vi "输入数据解析.vi"(0 "单个参数补充":dbl, 1 "从板号":dbl=1.0, 2 "主板二维码":string="BNET01", 3 "从板二维码":string="BNET01", 5 "主板引用":refnum<vi>, 7 "从板引用":refnum<vi>, 9 "主板选项":string="三级故障阀值", 11 "枚举":enum16{"主板", "从板"}(ring), 12 "快换":bool caption="快换写入") -> (4 "输出数组":dbl[][](array[numeric]), 6 "数组长度":dbl[](array[numeric]), 8 "循环次数":i32, 10 "命令":u32, 14 "名称":string[](array[string]), 15 "命令序号":u32[](array[numeric]))   [LabVIEW 2013] (continued)
                    n7569 = Quotient & Remainder(x=w19481, y=w19499) -> (x-y*floor(x/y)=w19498:dbl, floor(x/y)=w19502:dbl)
                    n7570 = Quotient & Remainder(x=w19480, y=w19494) -> (x-y*floor(x/y)=w19490:dbl, floor(x/y)=w19491:dbl)
                    n7571 = Quotient & Remainder(x=w19502, y=w19499) -> (x-y*floor(x/y)=w19497:dbl, floor(x/y)=w19501:dbl)
                    n7572 = Quotient & Remainder(x=w19491, y=w19494) -> (x-y*floor(x/y)=w19489:dbl, floor(x/y)=w19492:dbl)
                    n7573 = Quotient & Remainder(x=w19501, y=w19499) -> (x-y*floor(x/y)=w19496:dbl, floor(x/y)=w19500:dbl)
                    n7574 = Quotient & Remainder(x=w19492, y=w19494) -> (x-y*floor(x/y)=w19488:dbl, floor(x/y)=w19493:dbl)
                    n7575 = Quotient & Remainder(x=w19500, y=w19499) -> (x-y*floor(x/y)=w19495:dbl)  [unwired: 1 out]
                    n7576 = Quotient & Remainder(x=w19493, y=w19494) -> (x-y*floor(x/y)=w19487:dbl)  [unwired: 1 out]
                    n7577 = Build Array(w19495, w19496, w19497, w19498, w19487, w19488, w19489, w19490) -> (w19503:dbl[])
                  }
                  frame 3 {
                    w19511 = 256.0 ("y")
                    # "充电次数"
                    n7578 = Unbundle By Name(w19516) -> ("充电次数"=w19515:dbl, "应用车型"=w19513:dbl, "电池包组号"=w19512:dbl)
                    n7579 = Quotient & Remainder(x=w19515, y=w19511) -> (x-y*floor(x/y)=w19517:dbl, floor(x/y)=w19514:dbl)
                    n7580 = Quotient & Remainder(x=w19513, y=w19511) -> (x-y*floor(x/y)=w19509:dbl, floor(x/y)=w19510:dbl)
                    n7581 = Quotient & Remainder(x=w19512, y=w19511) -> (x-y*floor(x/y)=w19507:dbl, floor(x/y)=w19508:dbl)
                    n7582 = Build Array(w19514, w19517, w19510, w19509, w19508, w19507) -> (w19518:dbl[])
                  }
                  frame 4 {
                    # "SOC"
                    n7583 = Unbundle By Name(w19527) -> ("SOC"=w19526:dbl)
                    n7584 = call "输入分辨率计算-EV05.vi"("1字节?"=FALSE, "数值"=w19526, "分辨率"=0.1) -> ("低字节"=w19522:dbl, "高字节1"=w19523:dbl)  [unwired: 2 in, 5 out]
                    n7585 = Build Array(w19523, w19522) -> (w19528:dbl[])
                  }
                  frame 5 {
                    # "车牌号"
                    n7586 = Unbundle By Name(w19535) -> ("车牌号"=w19534:string)
                    n7587 = String To Byte Array(string=w19534) -> (unsigned byte array=w19538:u8[])
                    n7588 = Array Subset(array=w19538, length=8 ("长度")) -> (w19533:u8[])  [unwired: 1 in]
                  }
                  frame 6 {
                    n7589 = Unbundle By Name(w19556) -> ("最大允许单体电压"=w19554:dbl, "最大允许总电压"=w19553:dbl, "最大允许温度"=w19552:dbl, "最小允许温度"=w19551:dbl, "最大允许充电电流"=w19550:dbl, "最小允许充电电流"=w19549:dbl, "电流步长"=w19545:dbl, "最小允许单体电压"=w19548:dbl)
                    n7590 = call "输入分辨率计算-EV05.vi"("1字节?"=FALSE, "数值 2"=w19548, "数值"=w19554, "分辨率"=0.001) -> ("低字节 2"=w19540:dbl, "高字节 2"=w19541:dbl, "低字节"=w19564:dbl, "高字节1"=w19565:dbl)  [unwired: 1 in, 3 out]
                    n7591 = call "输入分辨率计算-EV05.vi"("1字节?"=FALSE, "数值"=w19553, "分辨率"=0.1) -> ("低字节"=w19562:dbl, "高字节1"=w19563:dbl)  [unwired: 2 in, 5 out]
                    n7592 = call "输入分辨率计算-EV05.vi"("1字节?"=TRUE, "数值 2"=w19551, "数值"=w19552, "偏移量"=-40.0, "分辨率"=1.0) -> ("高字节 2"=w19557:dbl, "高字节1"=w19561:dbl)  [unwired: 5 out]
                    n7593 = call "输入分辨率计算-EV05.vi"("1字节?"=FALSE, "数值 2"=w19549, "数值"=w19550, "偏移量"=0.0, "分辨率"=0.1) -> ("低字节 2"=w19546:dbl, "高字节 2"=w19547:dbl, "低字节"=w19559:dbl, "高字节1"=w19560:dbl)  [unwired: 3 out]
                    n7594 = Quotient & Remainder(x=w19545, y=256.0) -> (x-y*floor(x/y)=w19542:dbl, floor(x/y)=w19543:dbl)
                    n7595 = Build Array(w19565, w19564, w19563, w19562, w19561, w19557, w19560, w19559, w19547, w19546, w19543, w19542, w19541, w19540) -> (w19558:dbl[])
                  }
                }
              }
            }
          }
        }
        frame "电池包序号" {
          n7596 = case shown="真" w19580 {
            tunnel: [_ w19591] -> w19584
            tunnel: [_ w19590] -> w19583
            tunnel: w19582 -> [_ w19586]
            tunnel: [_ w19589] -> w19581
            tunnel: [_ u32 35 ("命令序号")] -> w19579
            frame False {
            }
            frame True {
              n7597 = Unbundle By Name(w19586) -> ("电池组信息(从板)"=w19587:refnum<vi>)
              n7598 = property class="Clust (严格)"(reference=w19587) -> ("Value"=w19585:T9)  [unwired: 1 in, 2 out]
              n7599 = for {
                N: 1 -> [_]
                tunnel: [w19597] -> w19591 mode=indexing
                tunnel: [w19596] -> w19590 mode=indexing
                tunnel: w19585 -> [w19595]
                tunnel: [w19594] -> w19589 mode=indexing
                i -> [w19593]
                n7600 = case shown="0, 默认" w19593 {
                  tunnel: [4 ("单个参数补充") 30 ("单个参数补充") 8 ("单个参数补充") 6 ("单个参数补充") 4 ("单个参数补充") 8 ("单个参数补充") 14 ("单个参数补充")] -> w19597
                  tunnel: [u32 2 ("命令序号") u32 1 ("命令序号") u32 3 ("命令序号") u32 4 ("命令序号") u32 5 ("命令序号") u32 6 ("命令序号") u32 7 ("命令序号")] -> w19596
                  tunnel: w19595 -> [w19605 w19621 w19633 w19662 w19672 w19679 w19699]
                  tunnel: [w19598 w19623 w19650 w19664 w19673 w19677 w19701] -> w19594
                  frame 0, Default {
                    n7601 = Unbundle By Name(w19605) -> ("电池包序号"=w19602:dbl)
                    n7602 = Quotient & Remainder(x=w19602, y=256.0) -> (x-y*floor(x/y)=w19599:dbl, floor(x/y)=w19600:dbl)
                    n7603 = Build Array(w19600, w19599) -> (w19598:dbl[])
                  }
                  frame 1 {
                    w19611 = 0 ("索引")
                    # "电池组信息"
                    n7604 = Unbundle By Name(w19621) -> ("电池类型"=w19613:dbl, "电池厂家"=w19612:dbl, "电池厂家"=w19614:dbl, "电池类型"=w19615:dbl, "额定能量"=w19619:dbl, "额定容量"=w19616:dbl, "实际容量"=w19608:dbl)
                    n7605 = Build Array(w19613, w19612, w19611, w19611, w19611, w19611, w19611, w19614, w19615) -> (w19610:dbl[])
                    n7606 = call "输入分辨率计算-EV05.vi"("1字节?"=FALSE, "数值"=w19608, "分辨率"=0.1) -> ("高字节1"=w19606:dbl)  [unwired: 2 in, 6 out]
                    n7607 = Quotient & Remainder(x=w19619, y=256.0) -> (x-y*floor(x/y)=w19617:dbl, floor(x/y)=w19618:dbl)
                    n7608 = call "电池组信息组合.vi"("数组"=w19610) -> ("电池信息组合"=w19624:dbl[])
                    n7609 = Insert Into Array(array=w19624, index=0 ("索引"), new element #1=w19618, new element #2=w19617, new element #3=w19616, new element #4=w19606, new element #5=w19606) -> (w19623:dbl[])
                  }
                  frame 2 {
                    w19641 = 256.0 ("y")
                    w19646 = 256.0 ("y")
                    # "充放电安时/安时数"
                    n7610 = Unbundle By Name(w19633) -> ("充电总安时"=w19630:dbl, "放电总这时"=w19629:dbl)
                    n7611 = call "输入分辨率计算-EV05.vi"("1字节?"=TRUE, "数值 2"=w19629, "数值"=w19630, "分辨率"=0.001) -> ("高字节 2"=w19627:dbl, "高字节1"=w19628:dbl)  [unwired: 1 in, 5 out]
                    n7612 = Quotient & Remainder(x=w19628, y=w19646) -> (x-y*floor(x/y)=w19645:dbl, floor(x/y)=w19649:dbl)
                    n7613 = Quotient & Remainder(x=w19627, y=w19641) -> (x-y*floor(x/y)=w19637:dbl, floor(x/y)=w19638:dbl)
                    n7614 = Quotient & Remainder(x=w19649, y=w19646) -> (x-y*floor(x/y)=w19644:dbl, floor(x/y)=w19648:dbl)
                    n7615 = Quotient & Remainder(x=w19638, y=w19641) -> (x-y*floor(x/y)=w19636:dbl, floor(x/y)=w19639:dbl)
                    n7616 = Quotient & Remainder(x=w19648, y=w19646) -> (x-y*floor(x/y)=w19643:dbl, floor(x/y)=w19647:dbl)
                    n7617 = Quotient & Remainder(x=w19639, y=w19641) -> (x-y*floor(x/y)=w19635:dbl, floor(x/y)=w19640:dbl)
                    n7618 = Quotient & Remainder(x=w19647, y=w19646) -> (x-y*floor(x/y)=w19642:dbl)  [unwired: 1 out]
                    n7619 = Quotient & Remainder(x=w19640, y=w19641) -> (x-y*floor(x/y)=w19634:dbl)  [unwired: 1 out]
                    n7620 = Build Array(w19642, w19643, w19644, w19645, w19634, w19635, w19636, w19637) -> (w19650:dbl[])
                  }
                  frame 3 {
                    w19657 = 256.0 ("y")
                    # "充电次数"
                    n7621 = Unbundle By Name(w19662) -> ("充电次数"=w19661:dbl, "应用车型"=w19659:dbl, "电池包组号"=w19658:dbl)
                    n7622 = Quotient & Remainder(x=w19661, y=w19657) -> (x-y*floor(x/y)=w19663:dbl, floor(x/y)=w19660:dbl)
                    n7623 = Quotient & Remainder(x=w19659, y=w19657) -> (x-y*floor(x/y)=w19655:dbl, floor(x/y)=w19656:dbl)
                    n7624 = Quotient & Remainder(x=w19658, y=w19657) -> (x-y*floor(x/y)=w19653:dbl, floor(x/y)=w19654:dbl)
                    n7625 = Build Array(w19660, w19663, w19656, w19655, w19654, w19653) -> (w19664:dbl[])
                  }
                  frame 4 {
                    # "SOC"
                    n7626 = Unbundle By Name(w19672) -> ("SOC"=w19671:dbl)
                    n7627 = call "输入分辨率计算-EV05.vi"("1字节?"=FALSE, "数值"=w19671, "分辨率"=0.1) -> ("低字节"=w19667:dbl, "高字节1"=w19668:dbl)  [unwired: 2 in, 5 out]
                    n7628 = Build Array(w19668, w19667) -> (w19673:dbl[])
                  }
                  frame 5 {
                    # "车牌号"
                    n7629 = Unbundle By Name(w19679) -> ("车牌号"=w19678:string)
                    n7630 = String To Byte Array(string=w19678) -> (unsigned byte array=w19682:u8[])
                    n7631 = Array Subset(array=w19682, length=8 ("长度")) -> (w19677:u8[])  [unwired: 1 in]
                  }
                  frame 6 {
                    n7632 = Unbundle By Name(w19699) -> ("最大允许单体电压"=w19697:dbl, "最大允许总电压"=w19696:dbl, "最大允许温度"=w19695:dbl, "最小允许温度"=w19694:dbl, "最大允许充电电流"=w19693:dbl, "最小允许充电电流"=w19692:dbl, "电流步长"=w19688:dbl, "最小允许单体电压"=w19691:dbl)
                    n7633 = call "输入分辨率计算-EV05.vi"("1字节?"=FALSE, "数值 2"=w19691, "数值"=w19697, "分辨率"=0.001) -> ("低字节 2"=w19683:dbl, "高字节 2"=w19684:dbl, "低字节"=w19707:dbl, "高字节1"=w19708:dbl)  [unwired: 1 in, 3 out]
                    n7634 = call "输入分辨率计算-EV05.vi"("1字节?"=FALSE, "数值"=w19696, "分辨率"=0.1) -> ("低字节"=w19705:dbl, "高字节1"=w19706:dbl)  [unwired: 2 in, 5 out]
                    n7635 = call "输入分辨率计算-EV05.vi"("1字节?"=TRUE, "数值 2"=w19694, "数值"=w19695, "偏移量"=-40.0, "分辨率"=1.0) -> ("高字节 2"=w19700:dbl, "高字节1"=w19704:dbl)  [unwired: 5 out]
                    n7636 = call "输入分辨率计算-EV05.vi"("1字节?"=FALSE, "数值 2"=w19692, "数值"=w19693, "偏移量"=0.0, "分辨率"=0.1) -> ("低字节 2"=w19689:dbl, "高字节 2"=w19690:dbl, "低字节"=w19702:dbl, "高字节1"=w19703:dbl)  [unwired: 3 out]
                    n7637 = Quotient & Remainder(x=w19688, y=256.0) -> (x-y*floor(x/y)=w19685:dbl, floor(x/y)=w19686:dbl)
                    n7638 = Build Array(w19708, w19707, w19706, w19705, w19704, w19700, w19703, w19702, w19690, w19689, w19686, w19685, w19684, w19683) -> (w19701:dbl[])
                  }
                }
              }
            }
          }
        }
        frame "充放电安时" {
          n7639 = case shown="真" w19723 {
            tunnel: [_ w19734] -> w19727
            tunnel: [_ w19733] -> w19726
            tunnel: w19725 -> [_ w19729]
            tunnel: [_ w19732] -> w19724
            tunnel: [_ u32 35 ("命令序号")] -> w19722
            frame False {
            }
            frame True {
              n7640 = Unbundle By Name(w19729) -> ("电池组信息(从板)"=w19730:refnum<vi>)
              n7641 = property class="Clust (严格)"(reference=w19730) -> ("Value"=w19728:T9)  [unwired: 1 in, 2 out]
              n7642 = for {
                N: 1 -> [_]
                tunnel: [w19740] -> w19734 mode=indexing
                tunnel: [w19739] -> w19733 mode=indexing
                tunnel: w19728 -> [w19738]
                tunnel: [w19737] -> w19732 mode=indexing
                i -> [w19736]
                n7643 = case shown="0, 默认" w19736 {
                  tunnel: [8 ("单个参数补充") 30 ("单个参数补充") 4 ("单个参数补充") 6 ("单个参数补充") 4 ("单个参数补充") 8 ("单个参数补充") 14 ("单个参数补充")] -> w19740
                  tunnel: [u32 3 ("命令序号") u32 1 ("命令序号") u32 2 ("命令序号") u32 4 ("命令序号") u32 5 ("命令序号") u32 6 ("命令序号") u32 7 ("命令序号")] -> w19739
                  tunnel: w19738 -> [w19747 w19782 w19795 w19805 w19815 w19822 w19842]
                  tunnel: [w19764 w19784 w19788 w19807 w19816 w19820 w19844] -> w19737
                  frame 0, Default {
                    w19755 = 256.0 ("y")
                    w19760 = 256.0 ("y")
                    # "充放电安时/安时数"
                    n7644 = Unbundle By Name(w19747) -> ("充电总安时"=w19744:dbl, "放电总这时"=w19743:dbl)
                    n7645 = call "输入分辨率计算-EV05.vi"("1字节?"=TRUE, "数值 2"=w19743, "数值"=w19744, "分辨率"=0.001) -> ("高字节 2"=w19741:dbl, "高字节1"=w19742:dbl)  [unwired: 1 in, 5 out]
                    n7646 = Quotient & Remainder(x=w19742, y=w19760) -> (x-y*floor(x/y)=w19759:dbl, floor(x/y)=w19763:dbl)
                    n7647 = Quotient & Remainder(x=w19741, y=w19755) -> (x-y*floor(x/y)=w19751:dbl, floor(x/y)=w19752:dbl)
                    n7648 = Quotient & Remainder(x=w19763, y=w19760) -> (x-y*floor(x/y)=w19758:dbl, floor(x/y)=w19762:dbl)
                    n7649 = Quotient & Remainder(x=w19752, y=w19755) -> (x-y*floor(x/y)=w19750:dbl, floor(x/y)=w19753:dbl)
                    n7650 = Quotient & Remainder(x=w19762, y=w19760) -> (x-y*floor(x/y)=w19757:dbl, floor(x/y)=w19761:dbl)
                    n7651 = Quotient & Remainder(x=w19753, y=w19755) -> (x-y*floor(x/y)=w19749:dbl, floor(x/y)=w19754:dbl)
                    n7652 = Quotient & Remainder(x=w19761, y=w19760) -> (x-y*floor(x/y)=w19756:dbl)  [unwired: 1 out]
                    n7653 = Quotient & Remainder(x=w19754, y=w19755) -> (x-y*floor(x/y)=w19748:dbl)  [unwired: 1 out]
                    n7654 = Build Array(w19756, w19757, w19758, w19759, w19748, w19749, w19750, w19751) -> (w19764:dbl[])
                  }
                  frame 1 {
                    w19772 = 0 ("索引")
                    # "电池组信息"
                    n7655 = Unbundle By Name(w19782) -> ("电池类型"=w19774:dbl, "电池厂家"=w19773:dbl, "电池厂家"=w19775:dbl, "电池类型"=w19776:dbl, "额定能量"=w19780:dbl, "额定容量"=w19777:dbl, "实际容量"=w19769:dbl)
                    n7656 = Build Array(w19774, w19773, w19772, w19772, w19772, w19772, w19772, w19775, w19776) -> (w19771:dbl[])
                    n7657 = call "输入分辨率计算-EV05.vi"("1字节?"=FALSE, "数值"=w19769, "分辨率"=0.1) -> ("高字节1"=w19767:dbl)  [unwired: 2 in, 6 out]
                    n7658 = Quotient & Remainder(x=w19780, y=256.0) -> (x-y*floor(x/y)=w19778:dbl, floor(x/y)=w19779:dbl)
                    n7659 = call "电池组信息组合.vi"("数组"=w19771) -> ("电池信息组合"=w19785:dbl[])
                    n7660 = Insert Into Array(array=w19785, index=0 ("索引"), new element #1=w19779, new element #2=w19778, new element #3=w19777, new element #4=w19767, new element #5=w19767) -> (w19784:dbl[])
                  }
                  frame 2 {
                    n7661 = Unbundle By Name(w19795) -> ("电池包序号"=w19792:dbl)
                    n7662 = Quotient & Remainder(x=w19792, y=256.0) -> (x-y*floor(x/y)=w19789:dbl, floor(x/y)=w19790:dbl)
                    n7663 = Build Array(w19790, w19789) -> (w19788:dbl[])
                  }
                  frame 3 {
                    w19800 = 256.0 ("y")
                    # "充电次数"
                    n7664 = Unbundle By Name(w19805) -> ("充电次数"=w19804:dbl, "应用车型"=w19802:dbl, "电池包组号"=w19801:dbl)
                    n7665 = Quotient & Remainder(x=w19804, y=w19800) -> (x-y*floor(x/y)=w19806:dbl, floor(x/y)=w19803:dbl)
                    n7666 = Quotient & Remainder(x=w19802, y=w19800) -> (x-y*floor(x/y)=w19798:dbl, floor(x/y)=w19799:dbl)
                    n7667 = Quotient & Remainder(x=w19801, y=w19800) -> (x-y*floor(x/y)=w19796:dbl, floor(x/y)=w19797:dbl)
                    n7668 = Build Array(w19803, w19806, w19799, w19798, w19797, w19796) -> (w19807:dbl[])
                  }
                  frame 4 {
                    # "SOC"
                    n7669 = Unbundle By Name(w19815) -> ("SOC"=w19814:dbl)
                    n7670 = call "输入分辨率计算-EV05.vi"("1字节?"=FALSE, "数值"=w19814, "分辨率"=0.1) -> ("低字节"=w19810:dbl, "高字节1"=w19811:dbl)  [unwired: 2 in, 5 out]
                    n7671 = Build Array(w19811, w19810) -> (w19816:dbl[])
                  }
                  frame 5 {
                    # "车牌号"
                    n7672 = Unbundle By Name(w19822) -> ("车牌号"=w19821:string)
                    n7673 = String To Byte Array(string=w19821) -> (unsigned byte array=w19825:u8[])
                    n7674 = Array Subset(array=w19825, length=8 ("长度")) -> (w19820:u8[])  [unwired: 1 in]
                  }
                  frame 6 {
                    n7675 = Unbundle By Name(w19842) -> ("最大允许单体电压"=w19840:dbl, "最大允许总电压"=w19839:dbl, "最大允许温度"=w19838:dbl, "最小允许温度"=w19837:dbl, "最大允许充电电流"=w19836:dbl, "最小允许充电电流"=w19835:dbl, "电流步长"=w19831:dbl, "最小允许单体电压"=w19834:dbl)
                    n7676 = call "输入分辨率计算-EV05.vi"("1字节?"=FALSE, "数值 2"=w19834, "数值"=w19840, "分辨率"=0.001) -> ("低字节 2"=w19826:dbl, "高字节 2"=w19827:dbl, "低字节"=w19850:dbl, "高字节1"=w19851:dbl)  [unwired: 1 in, 3 out]
                    n7677 = call "输入分辨率计算-EV05.vi"("1字节?"=FALSE, "数值"=w19839, "分辨率"=0.1) -> ("低字节"=w19848:dbl, "高字节1"=w19849:dbl)  [unwired: 2 in, 5 out]
                    n7678 = call "输入分辨率计算-EV05.vi"("1字节?"=TRUE, "数值 2"=w19837, "数值"=w19838, "偏移量"=-40.0, "分辨率"=1.0) -> ("高字节 2"=w19843:dbl, "高字节1"=w19847:dbl)  [unwired: 5 out]
                    n7679 = call "输入分辨率计算-EV05.vi"("1字节?"=FALSE, "数值 2"=w19835, "数值"=w19836, "偏移量"=0.0, "分辨率"=0.1) -> ("低字节 2"=w19832:dbl, "高字节 2"=w19833:dbl, "低字节"=w19845:dbl, "高字节1"=w19846:dbl)  [unwired: 3 out]
                    n7680 = Quotient & Remainder(x=w19831, y=256.0) -> (x-y*floor(x/y)=w19828:dbl, floor(x/y)=w19829:dbl)
                    n7681 = Build Array(w19851, w19850, w19849, w19848, w19847, w19843, w19846, w19845, w19833, w19832, w19829, w19828, w19827, w19826) -> (w19844:dbl[])
                  }
                }
              }
            }
          }
        }
        frame "充电次数时间" {
          n7682 = case shown="真" w19866 {
            tunnel: [_ w19877] -> w19870
            tunnel: [_ w19876] -> w19869
            tunnel: w19868 -> [_ w19872]
            tunnel: [_ w19875] -> w19867
            tunnel: [_ u32 35 ("命令序号")] -> w19865
            frame False {
            }
            frame True {
              n7683 = Unbundle By Name(w19872) -> ("电池组信息(从板)"=w19873:refnum<vi>)
              n7684 = property class="Clust (严格)"(reference=w19873) -> ("Value"=w19871:T9)  [unwired: 1 in, 2 out]
              n7685 = for {
                N: 1 -> [_]
                tunnel: [w19883] -> w19877 mode=indexing
                tunnel: [w19882] -> w19876 mode=indexing
                tunnel: w19871 -> [w19881]
                tunnel: [w19880] -> w19875 mode=indexing
                i -> [w19879]
                n7686 = case shown="0, 默认" w19879 {
                  tunnel: [6 ("单个参数补充") 30 ("单个参数补充") 4 ("单个参数补充") 8 ("单个参数补充") 4 ("单个参数补充") 8 ("单个参数补充") 14 ("单个参数补充")] -> w19883
                  tunnel: [u32 4 ("命令序号") u32 1 ("命令序号") u32 2 ("命令序号") u32 3 ("命令序号") u32 5 ("命令序号") u32 6 ("命令序号") u32 7 ("命令序号")] -> w19882
                  tunnel: w19881 -> [w19893 w19913 w19926 w19933 w19958 w19965 w19985]
                  tunnel: [w19895 w19915 w19919 w19950 w19959 w19963 w19987] -> w19880
                  frame 0, Default {
                    w19888 = 256.0 ("y")
                    # "充电次数"
                    n7687 = Unbundle By Name(w19893) -> ("放空次数"=w19892:dbl, "充满次数"=w19890:dbl, "充电次数"=w19889:dbl)
                    n7688 = Quotient & Remainder(x=w19892, y=w19888) -> (x-y*floor(x/y)=w19894:dbl, floor(x/y)=w19891:dbl)
                    n7689 = Quotient & Remainder(x=w19890, y=w19888) -> (x-y*floor(x/y)=w19886:dbl, floor(x/y)=w19887:dbl)
                    n7690 = Quotient & Remainder(x=w19889, y=w19888) -> (x-y*floor(x/y)=w19884:dbl, floor(x/y)=w19885:dbl)
                    n7691 = Build Array(w19891, w19894, w19887, w19886, w19885, w19884) -> (w19895:dbl[])
                  }
                  frame 1 {
                    w19903 = 0 ("索引")
                    # "电池组信息"
                    n7692 = Unbundle By Name(w19913) -> ("电池类型"=w19905:dbl, "电池厂家"=w19904:dbl, "电池厂家"=w19906:dbl, "电池类型"=w19907:dbl, "额定能量"=w19911:dbl, "额定容量"=w19908:dbl, "实际容量"=w19900:dbl)
                    n7693 = Build Array(w19905, w19904, w19903, w19903, w19903, w19903, w19903, w19906, w19907) -> (w19902:dbl[])
                    n7694 = call "输入分辨率计算-EV05.vi"("1字节?"=FALSE, "数值"=w19900, "分辨率"=0.1) -> ("高字节1"=w19898:dbl)  [unwired: 2 in, 6 out]
                    n7695 = Quotient & Remainder(x=w19911, y=256.0) -> (x-y*floor(x/y)=w19909:dbl, floor(x/y)=w19910:dbl)
                    n7696 = call "电池组信息组合.vi"("数组"=w19902) -> ("电池信息组合"=w19916:dbl[])
                    n7697 = Insert Into Array(array=w19916, index=0 ("索引"), new element #1=w19910, new element #2=w19909, new element #3=w19908, new element #4=w19898, new element #5=w19898) -> (w19915:dbl[])
                  }
                  frame 2 {
                    n7698 = Unbundle By Name(w19926) -> ("电池包序号"=w19923:dbl)
                    n7699 = Quotient & Remainder(x=w19923, y=256.0) -> (x-y*floor(x/y)=w19920:dbl, floor(x/y)=w19921:dbl)
                    n7700 = Build Array(w19921, w19920) -> (w19919:dbl[])
                  }
                  frame 3 {
                    w19941 = 256.0 ("y")
                    w19946 = 256.0 ("y")
                    # "充放电安时/安时数"
                    n7701 = Unbundle By Name(w19933) -> ("充电总安时"=w19930:dbl, "放电总这时"=w19929:dbl)
                    n7702 = call "输入分辨率计算-EV05.vi"("1字节?"=TRUE, "数值 2"=w19929, "数值"=w19930, "分辨率"=0.001) -> ("高字节 2"=w19927:dbl, "高字节1"=w19928:dbl)  [unwired: 1 in, 5 out]
                    n7703 = Quotient & Remainder(x=w19928, y=w19946) -> (x-y*floor(x/y)=w19945:dbl, floor(x/y)=w19949:dbl)
                    n7704 = Quotient & Remainder(x=w19927, y=w19941) -> (x-y*floor(x/y)=w19937:dbl, floor(x/y)=w19938:dbl)
                    n7705 = Quotient & Remainder(x=w19949, y=w19946) -> (x-y*floor(x/y)=w19944:dbl, floor(x/y)=w19948:dbl)
                    n7706 = Quotient & Remainder(x=w19938, y=w19941) -> (x-y*floor(x/y)=w19936:dbl, floor(x/y)=w19939:dbl)
                    n7707 = Quotient & Remainder(x=w19948, y=w19946) -> (x-y*floor(x/y)=w19943:dbl, floor(x/y)=w19947:dbl)
                    n7708 = Quotient & Remainder(x=w19939, y=w19941) -> (x-y*floor(x/y)=w19935:dbl, floor(x/y)=w19940:dbl)
                    n7709 = Quotient & Remainder(x=w19947, y=w19946) -> (x-y*floor(x/y)=w19942:dbl)  [unwired: 1 out]
                    n7710 = Quotient & Remainder(x=w19940, y=w19941) -> (x-y*floor(x/y)=w19934:dbl)  [unwired: 1 out]
                    n7711 = Build Array(w19942, w19943, w19944, w19945, w19934, w19935, w19936, w19937) -> (w19950:dbl[])
                  }
                  frame 4 {
                    # "SOC"
                    n7712 = Unbundle By Name(w19958) -> ("SOC"=w19957:dbl)
                    n7713 = call "输入分辨率计算-EV05.vi"("1字节?"=FALSE, "数值"=w19957, "分辨率"=0.1) -> ("低字节"=w19953:dbl, "高字节1"=w19954:dbl)  [unwired: 2 in, 5 out]
                    n7714 = Build Array(w19954, w19953) -> (w19959:dbl[])
                  }
                  frame 5 {
                    # "车牌号"
                    n7715 = Unbundle By Name(w19965) -> ("车牌号"=w19964:string)
                    n7716 = String To Byte Array(string=w19964) -> (unsigned byte array=w19968:u8[])
                    n7717 = Array Subset(array=w19968, length=8 ("长度")) -> (w19963:u8[])  [unwired: 1 in]
                  }
                  frame 6 {
                    n7718 = Unbundle By Name(w19985) -> ("最大允许单体电压"=w19983:dbl, "最大允许总电压"=w19982:dbl, "最大允许温度"=w19981:dbl, "最小允许温度"=w19980:dbl, "最大允许充电电流"=w19979:dbl, "最小允许充电电流"=w19978:dbl, "电流步长"=w19974:dbl, "最小允许单体电压"=w19977:dbl)
                    n7719 = call "输入分辨率计算-EV05.vi"("1字节?"=FALSE, "数值 2"=w19977, "数值"=w19983, "分辨率"=0.001) -> ("低字节 2"=w19969:dbl, "高字节 2"=w19970:dbl, "低字节"=w19993:dbl, "高字节1"=w19994:dbl)  [unwired: 1 in, 3 out]
                    n7720 = call "输入分辨率计算-EV05.vi"("1字节?"=FALSE, "数值"=w19982, "分辨率"=0.1) -> ("低字节"=w19991:dbl, "高字节1"=w19992:dbl)  [unwired: 2 in, 5 out]
                    n7721 = call "输入分辨率计算-EV05.vi"("1字节?"=TRUE, "数值 2"=w19980, "数值"=w19981, "偏移量"=-40.0, "分辨率"=1.0) -> ("高字节 2"=w19986:dbl, "高字节1"=w19990:dbl)  [unwired: 5 out]
                    n7722 = call "输入分辨率计算-EV05.vi"("1字节?"=FALSE, "数值 2"=w19978, "数值"=w19979, "偏移量"=0.0, "分辨率"=0.1) -> ("低字节 2"=w19975:dbl, "高字节 2"=w19976:dbl, "低字节"=w19988:dbl, "高字节1"=w19989:dbl)  [unwired: 3 out]
                    n7723 = Quotient & Remainder(x=w19974, y=256.0) -> (x-y*floor(x/y)=w19971:dbl, floor(x/y)=w19972:dbl)
                    n7724 = Build Array(w19994, w19993, w19992, w19991, w19990, w19986, w19989, w19988, w19976, w19975, w19972, w19971, w19970, w19969) -> (w19987:dbl[])
                  }
                }
              }
            }
          }
        }
        frame "SOC" {
          n7725 = case shown="真" w20009 {
            tunnel: [_ w20020] -> w20013
            tunnel: [_ w20019] -> w20012
            tunnel: w20011 -> [_ w20015]
            tunnel: [_ w20018] -> w20010
            tunnel: [_ u32 35 ("命令序号")] -> w20008
            frame False {
            }
            frame True {
              n7726 = Unbundle By Name(w20015) -> ("电池组信息(从板)"=w20016:refnum<vi>)
              n7727 = property class="Clust (严格)"(reference=w20016) -> ("Value"=w20014:T9)  [unwired: 1 in, 2 out]
              n7728 = for {
                N: 1 -> [_]
                tunnel: [w20026] -> w20020 mode=indexing
                tunnel: [w20025] -> w20019 mode=indexing
                tunnel: w20014 -> [w20024]
                tunnel: [w20023] -> w20018 mode=indexing
                i -> [w20022]
                n7729 = case shown="0, 默认" w20022 {
                  tunnel: [2 ("单个参数补充") 30 ("单个参数补充") 4 ("单个参数补充") 8 ("单个参数补充") 6 ("单个参数补充") 8 ("单个参数补充") 14 ("单个参数补充")] -> w20026
                  tunnel: [u32 5 ("命令序号") u32 1 ("命令序号") u32 2 ("命令序号") u32 3 ("命令序号") u32 4 ("命令序号") u32 6 ("命令序号") u32 7 ("命令序号")] -> w20025
                  tunnel: w20024 -> [w20032 w20051 w20064 w20071 w20100 w20108 w20128]
                  tunnel: [w20033 w20053 w20057 w20088 w20102 w20106 w20130] -> w20023
                  frame 0, Default {
                    # "SOC"
                    n7730 = Unbundle By Name(w20032) -> ("SOC"=w20031:dbl)
                    n7731 = call "输入分辨率计算-EV05.vi"("1字节?"=FALSE, "数值"=w20031, "分辨率"=0.1) -> ("低字节"=w20027:dbl, "高字节1"=w20028:dbl)  [unwired: 2 in, 5 out]
                    n7732 = Build Array(w20028, w20027) -> (w20033:dbl[])
                  }
                  frame 1 {
                    w20041 = 0 ("索引")
                    # "电池组信息"
                    n7733 = Unbundle By Name(w20051) -> ("电池类型"=w20043:dbl, "电池厂家"=w20042:dbl, "电池厂家"=w20044:dbl, "电池类型"=w20045:dbl, "额定能量"=w20049:dbl, "额定容量"=w20046:dbl, "实际容量"=w20038:dbl)
                    n7734 = Build Array(w20043, w20042, w20041, w20041, w20041, w20041, w20041, w20044, w20045) -> (w20040:dbl[])
                    n7735 = call "输入分辨率计算-EV05.vi"("1字节?"=FALSE, "数值"=w20038, "分辨率"=0.1) -> ("高字节1"=w20036:dbl)  [unwired: 2 in, 6 out]
                    n7736 = Quotient & Remainder(x=w20049, y=256.0) -> (x-y*floor(x/y)=w20047:dbl, floor(x/y)=w20048:dbl)
                    n7737 = call "电池组信息组合.vi"("数组"=w20040) -> ("电池信息组合"=w20054:dbl[])
                    n7738 = Insert Into Array(array=w20054, index=0 ("索引"), new element #1=w20048, new element #2=w20047, new element #3=w20046, new element #4=w20036, new element #5=w20036) -> (w20053:dbl[])
                  }
                  frame 2 {
                    n7739 = Unbundle By Name(w20064) -> ("电池包序号"=w20061:dbl)
                    n7740 = Quotient & Remainder(x=w20061, y=256.0) -> (x-y*floor(x/y)=w20058:dbl, floor(x/y)=w20059:dbl)
                    n7741 = Build Array(w20059, w20058) -> (w20057:dbl[])
                  }
                  frame 3 {
                    w20079 = 256.0 ("y")
                    w20084 = 256.0 ("y")
                    # "充放电安时/安时数"
                    n7742 = Unbundle By Name(w20071) -> ("充电总安时"=w20068:dbl, "放电总这时"=w20067:dbl)
                    n7743 = call "输入分辨率计算-EV05.vi"("1字节?"=TRUE, "数值 2"=w20067, "数值"=w20068, "分辨率"=0.001) -> ("高字节 2"=w20065:dbl, "高字节1"=w20066:dbl)  [unwired: 1 in, 5 out]
                    n7744 = Quotient & Remainder(x=w20066, y=w20084) -> (x-y*floor(x/y)=w20083:dbl, floor(x/y)=w20087:dbl)
                    n7745 = Quotient & Remainder(x=w20065, y=w20079) -> (x-y*floor(x/y)=w20075:dbl, floor(x/y)=w20076:dbl)
                    n7746 = Quotient & Remainder(x=w20087, y=w20084) -> (x-y*floor(x/y)=w20082:dbl, floor(x/y)=w20086:dbl)
                    n7747 = Quotient & Remainder(x=w20076, y=w20079) -> (x-y*floor(x/y)=w20074:dbl, floor(x/y)=w20077:dbl)
                    n7748 = Quotient & Remainder(x=w20086, y=w20084) -> (x-y*floor(x/y)=w20081:dbl, floor(x/y)=w20085:dbl)
                    n7749 = Quotient & Remainder(x=w20077, y=w20079) -> (x-y*floor(x/y)=w20073:dbl, floor(x/y)=w20078:dbl)
                    n7750 = Quotient & Remainder(x=w20085, y=w20084) -> (x-y*floor(x/y)=w20080:dbl)  [unwired: 1 out]
                    n7751 = Quotient & Remainder(x=w20078, y=w20079) -> (x-y*floor(x/y)=w20072:dbl)  [unwired: 1 out]
                    n7752 = Build Array(w20080, w20081, w20082, w20083, w20072, w20073, w20074, w20075) -> (w20088:dbl[])
                  }
                  frame 4 {
                    w20095 = 256.0 ("y")
                    # "充电次数"
                    n7753 = Unbundle By Name(w20100) -> ("充电次数"=w20099:dbl, "应用车型"=w20097:dbl, "电池包组号"=w20096:dbl)
                    n7754 = Quotient & Remainder(x=w20099, y=w20095) -> (x-y*floor(x/y)=w20101:dbl, floor(x/y)=w20098:dbl)
                    n7755 = Quotient & Remainder(x=w20097, y=w20095) -> (x-y*floor(x/y)=w20093:dbl, floor(x/y)=w20094:dbl)
                    n7756 = Quotient & Remainder(x=w20096, y=w20095) -> (x-y*floor(x/y)=w20091:dbl, floor(x/y)=w20092:dbl)
                    n7757 = Build Array(w20098, w20101, w20094, w20093, w20092, w20091) -> (w20102:dbl[])
                  }
                  frame 5 {
                    # "车牌号"
                    n7758 = Unbundle By Name(w20108) -> ("车牌号"=w20107:string)
                    n7759 = String To Byte Array(string=w20107) -> (unsigned byte array=w20111:u8[])
                    n7760 = Array Subset(array=w20111, length=8 ("长度")) -> (w20106:u8[])  [unwired: 1 in]
                  }
                  frame 6 {
                    n7761 = Unbundle By Name(w20128) -> ("最大允许单体电压"=w20126:dbl, "最大允许总电压"=w20125:dbl, "最大允许温度"=w20124:dbl, "最小允许温度"=w20123:dbl, "最大允许充电电流"=w20122:dbl, "最小允许充电电流"=w20121:dbl, "电流步长"=w20117:dbl, "最小允许单体电压"=w20120:dbl)
                    n7762 = call "输入分辨率计算-EV05.vi"("1字节?"=FALSE, "数值 2"=w20120, "数值"=w20126, "分辨率"=0.001) -> ("低字节 2"=w20112:dbl, "高字节 2"=w20113:dbl, "低字节"=w20136:dbl, "高字节1"=w20137:dbl)  [unwired: 1 in, 3 out]
                    n7763 = call "输入分辨率计算-EV05.vi"("1字节?"=FALSE, "数值"=w20125, "分辨率"=0.1) -> ("低字节"=w20134:dbl, "高字节1"=w20135:dbl)  [unwired: 2 in, 5 out]
                    n7764 = call "输入分辨率计算-EV05.vi"("1字节?"=TRUE, "数值 2"=w20123, "数值"=w20124, "偏移量"=-40.0, "分辨率"=1.0) -> ("高字节 2"=w20129:dbl, "高字节1"=w20133:dbl)  [unwired: 5 out]
                    n7765 = call "输入分辨率计算-EV05.vi"("1字节?"=FALSE, "数值 2"=w20121, "数值"=w20122, "偏移量"=0.0, "分辨率"=0.1) -> ("低字节 2"=w20118:dbl, "高字节 2"=w20119:dbl, "低字节"=w20131:dbl, "高字节1"=w20132:dbl)  [unwired: 3 out]
                    n7766 = Quotient & Remainder(x=w20117, y=256.0) -> (x-y*floor(x/y)=w20114:dbl, floor(x/y)=w20115:dbl)
                    n7767 = Build Array(w20137, w20136, w20135, w20134, w20133, w20129, w20132, w20131, w20119, w20118, w20115, w20114, w20113, w20112) -> (w20130:dbl[])
                  }
                }
              }
            }
          }
        }
        frame "车牌号" {
          n7768 = case shown="真" w20152 {
            tunnel: [_ w20163] -> w20156
            tunnel: [_ w20162] -> w20155
            tunnel: w20154 -> [_ w20158]
            tunnel: [_ w20161] -> w20153
            tunnel: [_ u32 35 ("命令序号")] -> w20151
            frame False {
            }
            frame True {
              n7769 = Unbundle By Name(w20158) -> ("电池组信息(从板)"=w20159:refnum<vi>)
              n7770 = property class="Clust (严格)"(reference=w20159) -> ("Value"=w20157:T9)  [unwired: 1 in, 2 out]
              n7771 = for {
                N: 1 -> [_]
                tunnel: [w20169] -> w20163 mode=indexing
                tunnel: [w20168] -> w20162 mode=indexing
                tunnel: w20157 -> [w20167]
                tunnel: [w20166] -> w20161 mode=indexing
                i -> [w20165]
                n7772 = case shown="0, 默认" w20165 {
                  tunnel: [8 ("单个参数补充") 30 ("单个参数补充") 4 ("单个参数补充") 8 ("单个参数补充") 6 ("单个参数补充") 4 ("单个参数补充") 14 ("单个参数补充")] -> w20169
                  tunnel: [u32 6 ("命令序号") u32 1 ("命令序号") u32 2 ("命令序号") u32 3 ("命令序号") u32 4 ("命令序号") u32 5 ("命令序号") u32 7 ("命令序号")] -> w20168
                  tunnel: w20167 -> [w20173 w20192 w20205 w20212 w20241 w20251 w20271]
                  tunnel: [w20171 w20194 w20198 w20229 w20243 w20252 w20273] -> w20166
                  frame 0, Default {
                    # "车牌号"
                    n7773 = Unbundle By Name(w20173) -> ("车牌号"=w20172:string)
                    n7774 = String To Byte Array(string=w20172) -> (unsigned byte array=w20176:u8[])
                    n7775 = Array Subset(array=w20176, length=8 ("长度")) -> (w20171:u8[])  [unwired: 1 in]
                  }
                  frame 1 {
                    w20182 = 0 ("索引")
                    # "电池组信息"
                    n7776 = Unbundle By Name(w20192) -> ("电池类型"=w20184:dbl, "电池厂家"=w20183:dbl, "电池厂家"=w20185:dbl, "电池类型"=w20186:dbl, "额定能量"=w20190:dbl, "额定容量"=w20187:dbl, "实际容量"=w20179:dbl)
                    n7777 = Build Array(w20184, w20183, w20182, w20182, w20182, w20182, w20182, w20185, w20186) -> (w20181:dbl[])
                    n7778 = call "输入分辨率计算-EV05.vi"("1字节?"=FALSE, "数值"=w20179, "分辨率"=0.1) -> ("高字节1"=w20177:dbl)  [unwired: 2 in, 6 out]
                    n7779 = Quotient & Remainder(x=w20190, y=256.0) -> (x-y*floor(x/y)=w20188:dbl, floor(x/y)=w20189:dbl)
                    n7780 = call "电池组信息组合.vi"("数组"=w20181) -> ("电池信息组合"=w20195:dbl[])
                    n7781 = Insert Into Array(array=w20195, index=0 ("索引"), new element #1=w20189, new element #2=w20188, new element #3=w20187, new element #4=w20177, new element #5=w20177) -> (w20194:dbl[])
                  }
                  frame 2 {
                    n7782 = Unbundle By Name(w20205) -> ("电池包序号"=w20202:dbl)
                    n7783 = Quotient & Remainder(x=w20202, y=256.0) -> (x-y*floor(x/y)=w20199:dbl, floor(x/y)=w20200:dbl)
                    n7784 = Build Array(w20200, w20199) -> (w20198:dbl[])
                  }
                  frame 3 {
                    w20220 = 256.0 ("y")
                    w20225 = 256.0 ("y")
                    # "充放电安时/安时数"
                    n7785 = Unbundle By Name(w20212) -> ("充电总安时"=w20209:dbl, "放电总这时"=w20208:dbl)
                    n7786 = call "输入分辨率计算-EV05.vi"("1字节?"=TRUE, "数值 2"=w20208, "数值"=w20209, "分辨率"=0.001) -> ("高字节 2"=w20206:dbl, "高字节1"=w20207:dbl)  [unwired: 1 in, 5 out]
                    n7787 = Quotient & Remainder(x=w20207, y=w20225) -> (x-y*floor(x/y)=w20224:dbl, floor(x/y)=w20228:dbl)
                    n7788 = Quotient & Remainder(x=w20206, y=w20220) -> (x-y*floor(x/y)=w20216:dbl, floor(x/y)=w20217:dbl)
                    n7789 = Quotient & Remainder(x=w20228, y=w20225) -> (x-y*floor(x/y)=w20223:dbl, floor(x/y)=w20227:dbl)
                    n7790 = Quotient & Remainder(x=w20217, y=w20220) -> (x-y*floor(x/y)=w20215:dbl, floor(x/y)=w20218:dbl)
                    n7791 = Quotient & Remainder(x=w20227, y=w20225) -> (x-y*floor(x/y)=w20222:dbl, floor(x/y)=w20226:dbl)
                    n7792 = Quotient & Remainder(x=w20218, y=w20220) -> (x-y*floor(x/y)=w20214:dbl, floor(x/y)=w20219:dbl)
                    n7793 = Quotient & Remainder(x=w20226, y=w20225) -> (x-y*floor(x/y)=w20221:dbl)  [unwired: 1 out]
                    n7794 = Quotient & Remainder(x=w20219, y=w20220) -> (x-y*floor(x/y)=w20213:dbl)  [unwired: 1 out]
                    n7795 = Build Array(w20221, w20222, w20223, w20224, w20213, w20214, w20215, w20216) -> (w20229:dbl[])
                  }
                  frame 4 {
                    w20236 = 256.0 ("y")
                    # "充电次数"
                    n7796 = Unbundle By Name(w20241) -> ("充电次数"=w20240:dbl, "应用车型"=w20238:dbl, "电池包组号"=w20237:dbl)
                    n7797 = Quotient & Remainder(x=w20240, y=w20236) -> (x-y*floor(x/y)=w20242:dbl, floor(x/y)=w20239:dbl)
                    n7798 = Quotient & Remainder(x=w20238, y=w20236) -> (x-y*floor(x/y)=w20234:dbl, floor(x/y)=w20235:dbl)
                    n7799 = Quotient & Remainder(x=w20237, y=w20236) -> (x-y*floor(x/y)=w20232:dbl, floor(x/y)=w20233:dbl)
                    n7800 = Build Array(w20239, w20242, w20235, w20234, w20233, w20232) -> (w20243:dbl[])
                  }
                  frame 5 {
                    # "SOC"
                    n7801 = Unbundle By Name(w20251) -> ("SOC"=w20250:dbl)
                    n7802 = call "输入分辨率计算-EV05.vi"("1字节?"=FALSE, "数值"=w20250, "分辨率"=0.1) -> ("低字节"=w20246:dbl, "高字节1"=w20247:dbl)  [unwired: 2 in, 5 out]
                    n7803 = Build Array(w20247, w20246) -> (w20252:dbl[])
                  }
                  frame 6 {
                    n7804 = Unbundle By Name(w20271) -> ("最大允许单体电压"=w20269:dbl, "最大允许总电压"=w20268:dbl, "最大允许温度"=w20267:dbl, "最小允许温度"=w20266:dbl, "最大允许充电电流"=w20265:dbl, "最小允许充电电流"=w20264:dbl, "电流步长"=w20260:dbl, "最小允许单体电压"=w20263:dbl)
                    n7805 = call "输入分辨率计算-EV05.vi"("1字节?"=FALSE, "数值 2"=w20263, "数值"=w20269, "分辨率"=0.001) -> ("低字节 2"=w20255:dbl, "高字节 2"=w20256:dbl, "低字节"=w20279:dbl, "高字节1"=w20280:dbl)  [unwired: 1 in, 3 out]
                    n7806 = call "输入分辨率计算-EV05.vi"("1字节?"=FALSE, "数值"=w20268, "分辨率"=0.1) -> ("低字节"=w20277:dbl, "高字节1"=w20278:dbl)  [unwired: 2 in, 5 out]
                    n7807 = call "输入分辨率计算-EV05.vi"("1字节?"=TRUE, "数值 2"=w20266, "数值"=w20267, "偏移量"=-40.0, "分辨率"=1.0) -> ("高字节 2"=w20272:dbl, "高字节1"=w20276:dbl)  [unwired: 5 out]
                    n7808 = call "输入分辨率计算-EV05.vi"("1字节?"=FALSE, "数值 2"=w20264, "数值"=w20265, "偏移量"=0.0, "分辨率"=0.1) -> ("低字节 2"=w20261:dbl, "高字节 2"=w20262:dbl, "低字节"=w20274:dbl, "高字节1"=w20275:dbl)  [unwired: 3 out]
                    n7809 = Quotient & Remainder(x=w20260, y=256.0) -> (x-y*floor(x/y)=w20257:dbl, floor(x/y)=w20258:dbl)
                    n7810 = Build Array(w20280, w20279, w20278, w20277, w20276, w20272, w20275, w20274, w20262, w20261, w20258, w20257, w20256, w20255) -> (w20273:dbl[])
                  }
                }
              }
            }
          }
        }
        frame "二维码" {
          w20303 = 30 ("长度")
          # "产品编号"
          n7811 = local read "从板二维码"() -> (w20292:string)
          n7812 = Search and Replace String(input string=w20292, search string="BNET" ("搜索字符串"), replace string="") -> (result string=w20298:string)  [unwired: 5 in, 3 out]
          n7813 = String To Byte Array(string=w20298) -> (unsigned byte array=w20301:u8[])
          n7814 = Array Subset(array=w20301, length=w20303) -> (w20305:u8[])  [unwired: 1 in]
          n7815 = Build Array(w20305) -> (w20297:u8[][])
          n7816 = Build Array(w20303) -> (w20295:i32[])
          n7817 = Build Array(u32 1 ("命令序号")) -> (w20294:u32[])
          n7818 = Build Array("写二维码") -> (w20296:string[])
        }
        frame "充电参数" {
          n7819 = case shown="真" w20310 {
            tunnel: [_ w20321] -> w20314
            tunnel: [_ w20320] -> w20313
            tunnel: w20312 -> [_ w20316]
            tunnel: [_ w20319] -> w20311
            tunnel: [_ u32 35 ("命令序号")] -> w20309
            frame False {
            }
            frame True {
              n7820 = Unbundle By Name(w20316) -> ("电池组信息(从板)"=w20317:refnum<vi>)
              n7821 = property class="Clust (严格)"(reference=w20317) -> ("Value"=w20315:T9)  [unwired: 1 in, 2 out]
              n7822 = for {
                N: 1 -> [_]
                tunnel: [w20327] -> w20321 mode=indexing
                tunnel: [w20326] -> w20320 mode=indexing
                tunnel: w20315 -> [w20325]
                tunnel: [w20324] -> w20319 mode=indexing
                i -> [w20323]
                n7823 = case shown="0, 默认" w20323 {
                  tunnel: [14 ("单个参数补充") 30 ("单个参数补充") 4 ("单个参数补充") 8 ("单个参数补充") 6 ("单个参数补充") 4 ("单个参数补充") 8 ("单个参数补充")] -> w20327
                  tunnel: [u32 7 ("命令序号") u32 1 ("命令序号") u32 2 ("命令序号") u32 3 ("命令序号") u32 4 ("命令序号") u32 5 ("命令序号") u32 6 ("命令序号")] -> w20326
                  tunnel: w20325 -> [w20344 w20380 w20393 w20400 w20429 w20439 w20446]
                  tunnel: [w20346 w20382 w20386 w20417 w20431 w20440 w20444] -> w20324
                  frame 0, Default {
                    n7824 = Unbundle By Name(w20344) -> ("最大允许单体电压"=w20342:dbl, "最大允许总电压"=w20341:dbl, "最大允许温度"=w20340:dbl, "最小允许温度"=w20339:dbl, "最大允许充电电流"=w20338:dbl, "最小允许充电电流"=w20337:dbl, "电流步长"=w20333:dbl, "最小允许单体电压"=w20336:dbl)
                    n7825 = call "输入分辨率计算-EV05.vi"("1字节?"=FALSE, "数值 2"=w20336, "数值"=w20342, "分辨率"=0.001) -> ("低字节 2"=w20328:dbl, "高字节 2"=w20329:dbl, "低字节"=w20352:dbl, "高字节1"=w20353:dbl)  [unwired: 1 in, 3 out]
                    n7826 = call "输入分辨率计算-EV05.vi"("1字节?"=FALSE, "数值"=w20341, "分辨率"=0.1) -> ("低字节"=w20350:dbl, "高字节1"=w20351:dbl)  [unwired: 2 in, 5 out]
                    n7827 = call "输入分辨率计算-EV05.vi"("1字节?"=TRUE, "数值 2"=w20339, "数值"=w20340, "偏移量"=-40.0, "分辨率"=1.0) -> ("高字节 2"=w20345:dbl, "高字节1"=w20349:dbl)  [unwired: 5 out]
                    n7828 = call "输入分辨率计算-EV05.vi"("1字节?"=FALSE, "数值 2"=w20337, "数值"=w20338, "偏移量"=0.0, "分辨率"=0.1) -> ("低字节 2"=w20334:dbl, "高字节 2"=w20335:dbl, "低字节"=w20347:dbl, "高字节1"=w20348:dbl)  [unwired: 3 out]
                    n7829 = Quotient & Remainder(x=w20333, y=256.0) -> (x-y*floor(x/y)=w20330:dbl, floor(x/y)=w20331:dbl)
                    n7830 = Build Array(w20353, w20352, w20351, w20350, w20349, w20345, w20348, w20347, w20335, w20334, w20331, w20330, w20329, w20328) -> (w20346:dbl[])
                  }
                  frame 1 {
                    w20370 = 0 ("索引")
                    # "电池组信息"
                    n7831 = Unbundle By Name(w20380) -> ("电池类型"=w20372:dbl, "电池厂家"=w20371:dbl, "电池厂家"=w20373:dbl, "电池类型"=w20374:dbl, "额定能量"=w20378:dbl, "额定容量"=w20375:dbl, "实际容量"=w20367:dbl)
                    n7832 = Build Array(w20372, w20371, w20370, w20370, w20370, w20370, w20370, w20373, w20374) -> (w20369:dbl[])
                    n7833 = call "输入分辨率计算-EV05.vi"("1字节?"=FALSE, "数值"=w20367, "分辨率"=0.1) -> ("高字节1"=w20365:dbl)  [unwired: 2 in, 6 out]
                    n7834 = Quotient & Remainder(x=w20378, y=256.0) -> (x-y*floor(x/y)=w20376:dbl, floor(x/y)=w20377:dbl)
                    n7835 = call "电池组信息组合.vi"("数组"=w20369) -> ("电池信息组合"=w20383:dbl[])
                    n7836 = Insert Into Array(array=w20383, index=0 ("索引"), new element #1=w20377, new element #2=w20376, new element #3=w20375, new element #4=w20365, new element #5=w20365) -> (w20382:dbl[])
                  }
                  frame 2 {
                    n7837 = Unbundle By Name(w20393) -> ("电池包序号"=w20390:dbl)
                    n7838 = Quotient & Remainder(x=w20390, y=256.0) -> (x-y*floor(x/y)=w20387:dbl, floor(x/y)=w20388:dbl)
                    n7839 = Build Array(w20388, w20387) -> (w20386:dbl[])
                  }
                  frame 3 {
                    w20408 = 256.0 ("y")
                    w20413 = 256.0 ("y")
                    # "充放电安时/安时数"
                    n7840 = Unbundle By Name(w20400) -> ("充电总安时"=w20397:dbl, "放电总这时"=w20396:dbl)
                    n7841 = call "输入分辨率计算-EV05.vi"("1字节?"=TRUE, "数值 2"=w20396, "数值"=w20397, "分辨率"=0.001) -> ("高字节 2"=w20394:dbl, "高字节1"=w20395:dbl)  [unwired: 1 in, 5 out]
                    n7842 = Quotient & Remainder(x=w20395, y=w20413) -> (x-y*floor(x/y)=w20412:dbl, floor(x/y)=w20416:dbl)
                    n7843 = Quotient & Remainder(x=w20394, y=w20408) -> (x-y*floor(x/y)=w20404:dbl, floor(x/y)=w20405:dbl)
                    n7844 = Quotient & Remainder(x=w20416, y=w20413) -> (x-y*floor(x/y)=w20411:dbl, floor(x/y)=w20415:dbl)
                    n7845 = Quotient & Remainder(x=w20405, y=w20408) -> (x-y*floor(x/y)=w20403:dbl, floor(x/y)=w20406:dbl)
                    n7846 = Quotient & Remainder(x=w20415, y=w20413) -> (x-y*floor(x/y)=w20410:dbl, floor(x/y)=w20414:dbl)
                    n7847 = Quotient & Remainder(x=w20406, y=w20408) -> (x-y*floor(x/y)=w20402:dbl, floor(x/y)=w20407:dbl)
                    n7848 = Quotient & Remainder(x=w20414, y=w20413) -> (x-y*floor(x/y)=w20409:dbl)  [unwired: 1 out]
                    n7849 = Quotient & Remainder(x=w20407, y=w20408) -> (x-y*floor(x/y)=w20401:dbl)  [unwired: 1 out]
                    n7850 = Build Array(w20409, w20410, w20411, w20412, w20401, w20402, w20403, w20404) -> (w20417:dbl[])
                  }
                  frame 4 {
                    w20424 = 256.0 ("y")
                    # "充电次数"
                    n7851 = Unbundle By Name(w20429) -> ("充电次数"=w20428:dbl, "应用车型"=w20426:dbl, "电池包组号"=w20425:dbl)
                    n7852 = Quotient & Remainder(x=w20428, y=w20424) -> (x-y*floor(x/y)=w20430:dbl, floor(x/y)=w20427:dbl)
                    n7853 = Quotient & Remainder(x=w20426, y=w20424) -> (x-y*floor(x/y)=w20422:dbl, floor(x/y)=w20423:dbl)
                    n7854 = Quotient & Remainder(x=w20425, y=w20424) -> (x-y*floor(x/y)=w20420:dbl, floor(x/y)=w20421:dbl)
                    n7855 = Build Array(w20427, w20430, w20423, w20422, w20421, w20420) -> (w20431:dbl[])
                  }
                  frame 5 {
                    # "SOC"
                    n7856 = Unbundle By Name(w20439) -> ("SOC"=w20438:dbl)
                    n7857 = call "输入分辨率计算-EV05.vi"("1字节?"=FALSE, "数值"=w20438, "分辨率"=0.1) -> ("低字节"=w20434:dbl, "高字节1"=w20435:dbl)  [unwired: 2 in, 5 out]
                    n7858 = Build Array(w20435, w20434) -> (w20440:dbl[])
                  }
                  frame 6 {
                    # "车牌号"
                    n7859 = Unbundle By Name(w20446) -> ("车牌号"=w20445:string)
                    n7860 = String To Byte Array(string=w20445) -> (unsigned byte array=w20449:u8[])
                    n7861 = Array Subset(array=w20449, length=8 ("长度")) -> (w20444:u8[])  [unwired: 1 in]
                  }
                }
              }
            }
          }
        }
      }
    }
  }
  "输出数组" <- w9
  "命令序号" <- w8
  "数组长度" <- w7
  "命令" <- w6
  "循环次数" <- w2
  "名称" <- w1
